vi "Analog Input And Output.vi"() -> ()   [LabVIEW 2012]
uses:
  <vilib>/DAQmx/read.llb/DAQmx Read (Analog DBL 1Chan 1Samp).vi
  <vilib>/DAQmx/write.llb/DAQmx Write (Analog DBL 1Chan 1Samp).vi
  <vilib>/DAQmx/create/channels.llb/DAQmx Create Channel (AI-Voltage-Basic).vi
  <vilib>/DAQmx/create/channels.llb/DAQmx Create Channel (AO-Voltage-Basic).vi
  <vilib>/DAQmx/miscellaneous.llb/DAQmx Fill In Error Info.vi
panel:
  in  "physical channels 2":tag
  in  "physical channels":tag
  out "Voltage":dbl
  in  "?":bool
  # "Analog I/O Program"
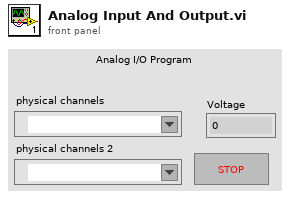
[diagram p1: front panel]
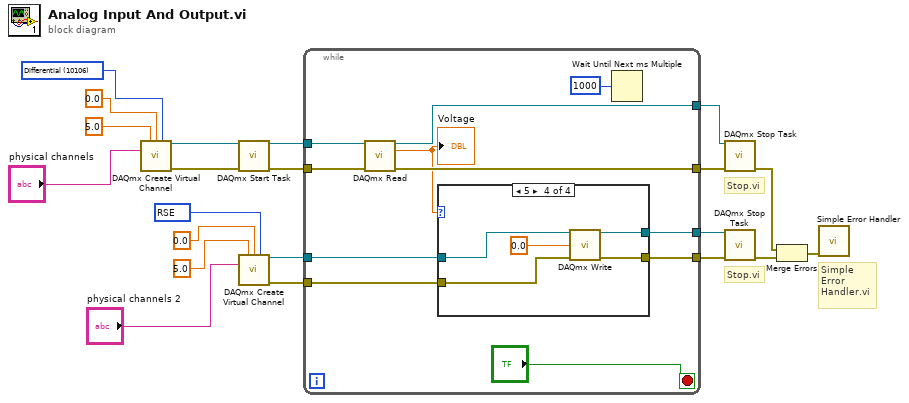
[diagram p0: block diagram]
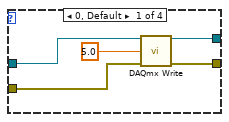
[diagram p2: hidden frame]
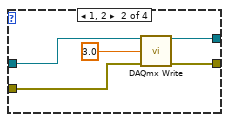
[diagram p3: hidden frame]
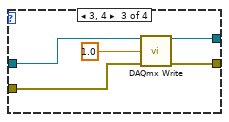
[diagram p4: hidden frame]
diagram:
  w12 = 10083 items=["Default"=-1, "RSE"=10083, "Differential"=10106, "Pseudodifferential"=12529] ("output terminal configuration")
  w15 = 10106 items=["default"=-1, "RSE"=10083, "NRSE"=10078, "Differential"=10106, "Pseudodifferential"=12529] ("input terminal configuration")
  # "Stop.vi"
  # "Simple\nError\nHandler.vi"
  # "Stop.vi"
  n1 = call-poly <vilib>:"DAQmx Create Virtual Channel.vi"("maximum value"=5.0, "minimum value"=0.0, "input terminal configuration"=w15, "physical channels"="physical channels") -> ("task out"=w13:refnum<k21>, "error out"=w14:errorcluster)  [unwired: 10 in]
  n2 = call <vilib>:"DAQmx Start Task.vi"("task/channels in"=w13, "error in"=w14) -> ("task out"=w16:refnum<k21>, "error out"=w17:errorcluster)  [unwired: 12 in]
  n3 = call-poly <vilib>:"DAQmx Create Virtual Channel.vi"("maximum value"=5.0, "minimum value"=0.0, "output terminal configuration"=w12, "physical channels"="physical channels 2") -> ("task out"=w20:refnum<k21>, "error out"=w21:errorcluster)  [unwired: 10 in]
  n4 = while {
    tunnel: w16 -> [w32]
    tunnel: w17 -> [w31]
    tunnel: [w30] -> w18
    tunnel: [w29] -> w19
    tunnel: w20 -> [w25]
    tunnel: w21 -> [w24]
    tunnel: [w23] -> w4
    tunnel: [w22] -> w3
    stop <- "?" stop-if-true
    n5 = call-poly <vilib>:"DAQmx Read.vi"("task/channels in"=w32, "error in"=w31) -> ("task out"=w30:refnum<k21>, "data"=w26:dbl, "error out"=w29:errorcluster)  [unwired: 11 in]
    "Voltage" <- w26
    n6 = case shown="5" w26 {
      tunnel: w25 -> [w37 w42 w47 w52]
      tunnel: w24 -> [w36 w41 w46 w51]
      tunnel: [w34 w39 w44 w48] -> w23
      tunnel: [w33 w38 w43 w49] -> w22
      frame 0, Default {
        n7 = call-poly <vilib>:"DAQmx Write.vi"("task/channels in"=w37, "data"=5.0, "error in"=w36) -> ("task out"=w34:refnum<k21>, "error out"=w33:errorcluster)  [unwired: 10 in, 1 out]
      }
      frame 1, 2 {
        n8 = call-poly <vilib>:"DAQmx Write.vi"("task/channels in"=w42, "data"=3.0, "error in"=w41) -> ("task out"=w39:refnum<k21>, "error out"=w38:errorcluster)  [unwired: 10 in, 1 out]
      }
      frame 3, 4 {
        n9 = call-poly <vilib>:"DAQmx Write.vi"("task/channels in"=w47, "data"=1.0, "error in"=w46) -> ("task out"=w44:refnum<k21>, "error out"=w43:errorcluster)  [unwired: 10 in, 1 out]
      }
      frame 5 {
        n10 = call-poly <vilib>:"DAQmx Write.vi"("task/channels in"=w52, "data"=0.0, "error in"=w51) -> ("task out"=w48:refnum<k21>, "error out"=w49:errorcluster)  [unwired: 10 in, 1 out]
      }
    }
    n11 = Wait Until Next ms Multiple(millisecond multiple=u32 1000) -> ()  [unwired: 1 out]
  }
  n12 = call <vilib>:"DAQmx Stop Task.vi"("task/channels in"=w18, "error in"=w19) -> ("error out"=w11:errorcluster)  [unwired: 12 in, 1 out]
  n13 = call <vilib>:"DAQmx Stop Task.vi"("task/channels in"=w4, "error in"=w3) -> ("error out"=w10:errorcluster)  [unwired: 12 in, 1 out]
  n14 = Merge Errors(w11, w10) -> (w9:errorcluster)
  n15 = call <vilib>:"Simple Error Handler.vi"("error in (no error)"=w9) -> ()  [unwired: 4 in, 5 out]
